vi "DriveForDistanceController.vi"(0 "Distance":dbl=60.0, 5 "Angle":dbl, 9 "SensorData":T2={"LeftDistance"=6.5916152770030445, "RightDistance"=6.599641480142774, "LeftVelocity"=46.58677937827863, "RightVelocity"=46.493891086439575, "Angle"=-0.015328918847370969, "Location"={6.595627830179985, 0.002635162832215609}}, 11 "Gains":T1={"FFV"=0.0055, "FFA"=0.0025, "Vel PID"={"P"=0.005, "I"=0.0, "D"=0.0}}, 12 "Trackwidth":dbl=30.0 format="%#_13g", 13 "Reset":bool) -> (4 "Left Speed":dbl=0.7370843765433353, 6 "Right Speed":dbl=0.7364472908610777, 10 "Done":bool, 14 "Graph":cluster{cluster{"x":dbl, "y":dbl}[]}[](graph)=[{[{"x"=0.0, "y"=0.0}, {"x"=6.0, "y"=0.0}, {"x"=12.0, "y"=0.0}, {"x"=18.0, "y"=0.0}, {"x"=24.0, "y"=0.0}, {"x"=30.0, "y"=0.0}, {"x"=36.0, "y"=0.0}, {"x"=42.0, "y"=0.0}, {"x"=48.0, "y"=0.0}, {"x"=54.0, "y"=0.0}, {"x"=55.0, "y"=0.0}, {"x"=60.0, "y"=0.0}]}, {[{"x"=6.595627830179985, "y"=0.002635162832215609}, {"x"=18.59562740071374, "y"=0.005845644049807444}]}, {[{"x"=18.595627540843186, "y"=0.0}]}, {[{"x"=18.595627830179986, "y"=0.002635162832215609}, {"x"=18.333399038985654, "y"=2.4975754526453273}, {"x"=17.558173321891196, "y"=4.883474879741818}, {"x"=16.303831762679355, "y"=7.0560581903418935}, {"x"=14.625195106486284, "y"=8.920373068560945}, {"x"=12.595627830179986, "y"=10.394940008245479}, {"x"=10.303831762679355, "y"=11.415313358374057}, {"x"=7.849969389391829, "y"=11.936897907251494}, {"x"=5.341286270968144, "y"=11.936897907251495}, {"x"=2.8874238976806166, "y"=11.415313358374059}, {"x"=0.5956278301799873, "y"=10.394940008245479}, {"x"=-1.4339394461263106, "y"=8.920373068560949}, {"x"=-3.112576102319383, "y"=7.056058190341894}, {"x"=-4.366917661531224, "y"=4.883474879741821}, {"x"=-5.142143378625682, "y"=2.497575452645332}, {"x"=-5.404372169820015, "y"=0.0026351628322170786}, {"x"=-5.142143378625684, "y"=-2.4923051269808933}, {"x"=-4.366917661531228, "y"=-4.878204554077382}, {"x"=-3.1125761023193865, "y"=-7.050787864677461}, {"x"=-1.4339394461263177, "y"=-8.915102742896513}, {"x"=0.5956278301799793, "y"=-10.389669682581046}, {"x"=2.887423897680614, "y"=-11.410043032709627}, {"x"=5.3412862709681335, "y"=-11.931627581587064}, {"x"=7.849969389391821, "y"=-11.931627581587065}, {"x"=10.303831762679351, "y"=-11.410043032709629}, {"x"=12.595627830179977, "y"=-10.389669682581053}, {"x"=14.625195106486277, "y"=-8.91510274289652}, {"x"=16.30383176267935, "y"=-7.050787864677464}, {"x"=17.558173321891193, "y"=-4.878204554077395}, {"x"=18.33339903898565, "y"=-2.492305126980903}, {"x"=18.595627830179986, "y"=0.00263516283221267}]}, {[{"x"=12326.754773558361, "y"=-12316.860814743844}, {"x"=12057.601746111126, "y"=-9756.040817653475}, {"x"=11261.905942608384, "y"=-7307.140942613652}, {"x"=9974.443087835292, "y"=-5077.189865288984}, {"x"=8251.481486477638, "y"=-3163.647148251028}, {"x"=6168.322828201805, "y"=-1650.1437904310478}, {"x"=3816.0111424787337, "y"=-602.8271511606581}, {"x"=1297.3537376183413, "y"=-67.46999315879293}, {"x"=-1277.571971927846, "y"=-67.46999315879111}, {"x"=-3796.2293767882416, "y"=-602.8271511606563}, {"x"=-6148.541062511309, "y"=-1650.143790431046}, {"x"=-8231.699720787143, "y"=-3163.647148251024}, {"x"=-9954.661322144799, "y"=-5077.189865288982}, {"x"=-11242.12417691789, "y"=-7307.14094261365}, {"x"=-12037.819980420634, "y"=-9756.04081765347}, {"x"=-12306.97300786787, "y"=-12316.860814743843}, {"x"=-12037.819980420634, "y"=-14877.68081183421}, {"x"=-11242.124176917896, "y"=-17326.580686874033}, {"x"=-9954.6613221448, "y"=-19556.531764198706}, {"x"=-8231.69972078715, "y"=-21470.07448123666}, {"x"=-6148.541062511317, "y"=-22983.57783905664}, {"x"=-3796.2293767882443, "y"=-24030.89447832703}, {"x"=-1277.5719719278572, "y"=-24566.251636328896}, {"x"=1297.3537376183326, "y"=-24566.251636328896}, {"x"=3816.011142478731, "y"=-24030.894478327034}, {"x"=6168.322828201795, "y"=-22983.57783905665}, {"x"=8251.481486477633, "y"=-21470.07448123667}, {"x"=9974.44308783529, "y"=-19556.531764198706}, {"x"=11261.90594260838, "y"=-17326.580686874047}, {"x"=12057.601746111126, "y"=-14877.68081183422}, {"x"=12326.754773558361, "y"=-12316.860814743848}]}], 15 "Time Left":dbl=20.0)   [LabVIEW 2019]
uses:
  PurePursuit/RobotNeededPathData.ctl
panel:
  in  "MaxDeAccel":dbl=120.0 format="%#_13g"
  in  "LookaheadDist":dbl=20.0
  in  "SlowSpeed":dbl=23.0 format="%#_13g"
  in  "SlowDistanceAtEnd":dbl=12.0 format="%#_13g"
  in  "MaxAccel":dbl=100.0
  in  "MaxVel":dbl=60.0
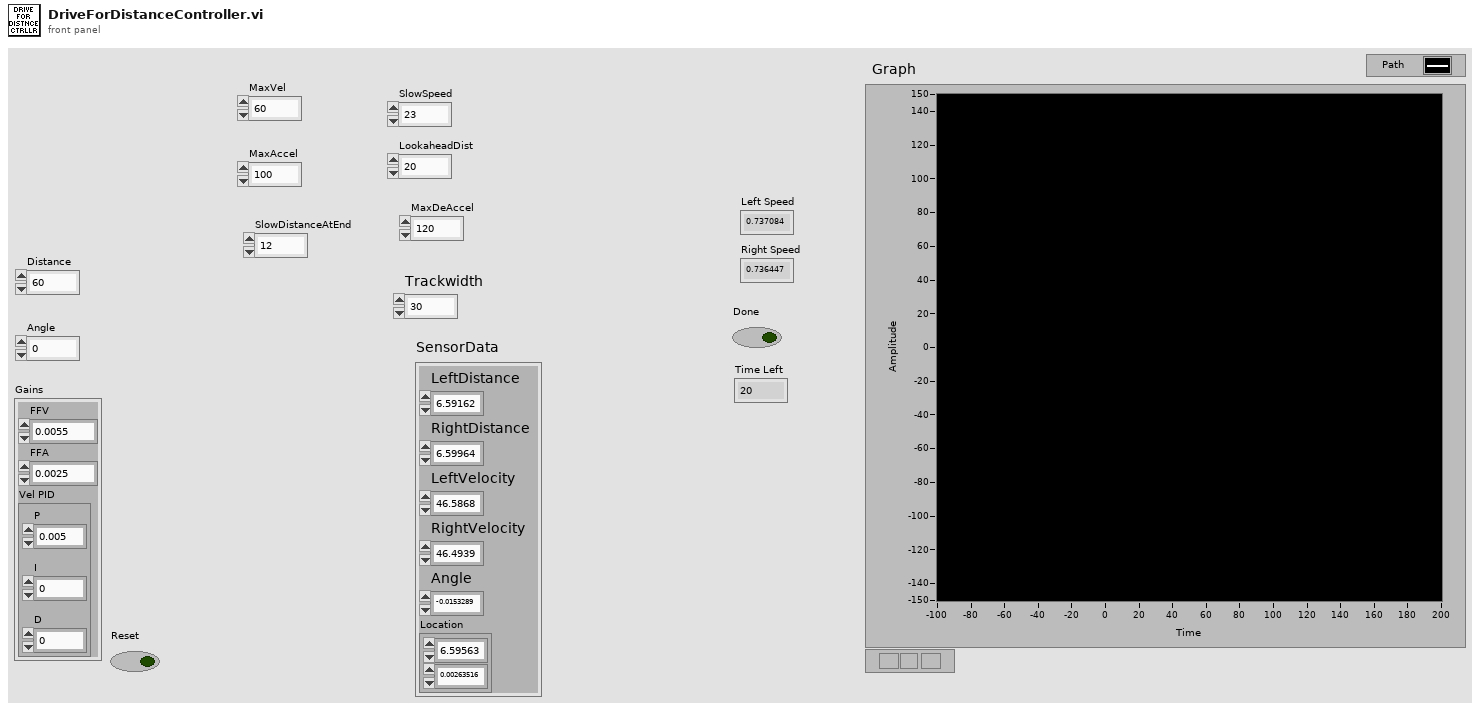
[diagram p1: front panel]
types:
  T1 = cluster{"FFV":dbl, "FFA":dbl, "Vel PID":cluster{"P":dbl, "I":dbl, "D":dbl}}
  T2 = cluster{"LeftDistance":dbl, "RightDistance":dbl, "LeftVelocity":dbl, "RightVelocity":dbl, "Angle":dbl, "Location":cluster{dbl, dbl}}
  T3 = typedef "RobotNeededPathData.ctl" = cluster{"Path":cluster{dbl, dbl}[], "MaxVel":dbl, "MaxAccel":dbl, "Backwards?":bool, "PointSpacing":dbl, "LookaheadDist":dbl, "Speed/Curve":dbl, "SlowDistanceAtEnd":dbl, "SlowSpeed":dbl, "MaxDeAccel":dbl}
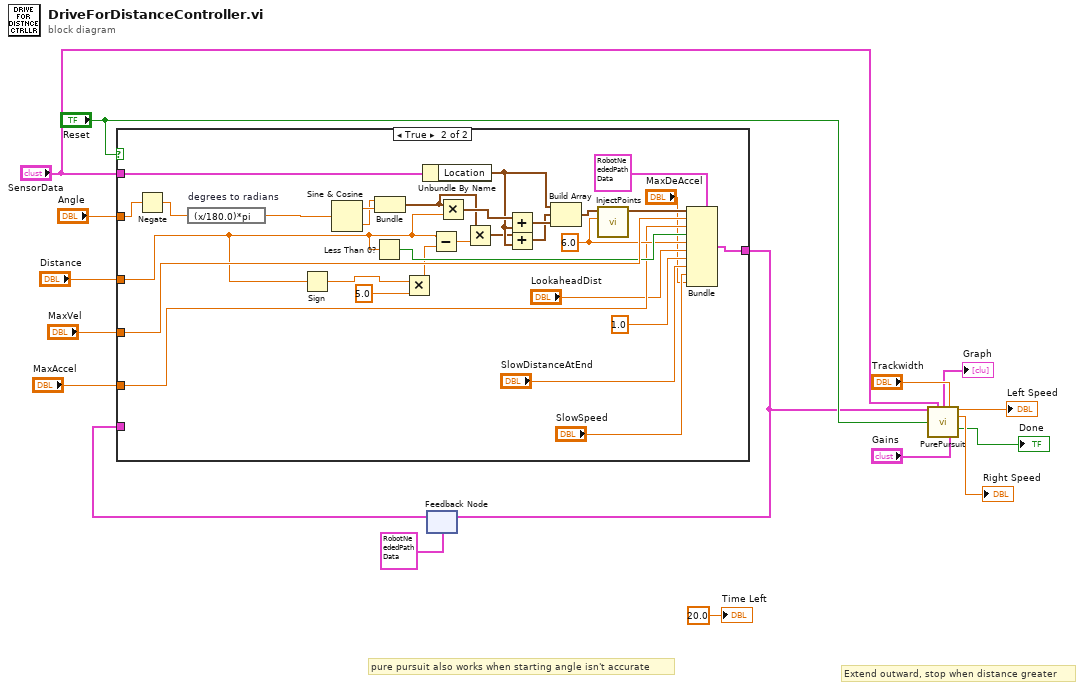
[diagram p0: block diagram]
diagram:
  # "pure pursuit also works when starting angle isn't accurate"
  # "Extend outward, stop when distance greater"
  n1 = feedback #1(T3 {"Path"=[], "MaxVel"=0.0, "MaxAccel"=0.0, "Backwards?"=FALSE, "PointSpacing"=0.0, "LookaheadDist"=0.0, "Speed/Curve"=1.8, "SlowDistanceAtEnd"=12.0, "SlowSpeed"=15.0, "MaxDeAccel"=0.0} ("RobotNeededPathData")) -> (w8:T3)
  n2 = case shown="True" "Reset" {
    tunnel: "SensorData" -> [_ w47]
    tunnel: "Angle" -> [_ w30]
    tunnel: "Distance" -> [_ w21]
    tunnel: "MaxVel" -> [_ w39]
    tunnel: "MaxAccel" -> [_ w35]
    tunnel: [w17 w31] -> w6
    tunnel: w8 -> [w17 _]
    frame False {
    }
    frame True {
      w37 = 6.0 ("Spacing")
      n3 = Negate(x=w30) -> (-x=w29:dbl)
      n4 = expression code="(x/180.0)*pi" "degrees to radians"(w29) -> (w46:dbl)
      n5 = Sign(1:w21) -> (0:w22:dbl)
      n6 = Sine & Cosine(0:w46) -> (1:w45:dbl, 2:w44:dbl)
      n7 = Less Than 0?(x=w21) -> (x < 0?=w38:bool)
      n8 = Bundle(w44, w45) -> (w28:cluster{dbl, dbl})  [unwired: 1 in]
      n9 = Multiply(x=w22, y=5.0) -> (x*y=w20:dbl)
      n10 = Unbundle By Name(w47) -> ("Location"=w27:cluster{dbl, dbl})
      n11 = Subtract(x=w21, y=w20) -> (x-y=w25:dbl)
      n12 = Multiply(x=w28, y=w21) -> (x*y=w43:cluster{dbl, dbl})
      n13 = Multiply(x=w28, y=w25) -> (x*y=w26:cluster{dbl, dbl})
      n14 = Add(x=w43, y=w27) -> (x+y=w19:cluster{dbl, dbl})
      n15 = Add(x=w26, y=w27) -> (x+y=w18:cluster{dbl, dbl})
      n16 = Build Array(w27, w18, w19) -> (w42:cluster{dbl, dbl}[])
      n17 = call "InjectPoints.vi"("Spacing"=w37, "Path"=w42) -> ("Path out"=w40:cluster{dbl, dbl}[])  [unwired: 9 in]
      n18 = Bundle(cluster=T3 {"Path"=[], "MaxVel"=0.0, "MaxAccel"=0.0, "Backwards?"=FALSE, "PointSpacing"=0.0, "LookaheadDist"=0.0, "Speed/Curve"=1.8, "SlowDistanceAtEnd"=12.0, "SlowSpeed"=15.0, "MaxDeAccel"=0.0} ("RobotNeededPathData"), "Path"=w40, "MaxVel"=w39, "MaxAccel"=w35, "Backwards?"=w38, "PointSpacing"=w37, "LookaheadDist"="LookaheadDist", "Speed/Curve"=1.0, "SlowDistanceAtEnd"="SlowDistanceAtEnd", "SlowSpeed"="SlowSpeed", "MaxDeAccel"="MaxDeAccel") -> (w31:T3)
    }
  }
  n19 = feedback-in #1(w6) -> ()
  n20 = call "PurePursuit.vi"("RobotNeededPathData"=w6, "SensorData"="SensorData", "Trackwidth"="Trackwidth", "Reset"="Reset", "Gains"="Gains") -> ("Graph"=→"Graph":cluster{cluster{"x":dbl, "y":dbl}[]}[], "LeftValue"=→"Left Speed":dbl, "RightValue"=→"Right Speed":dbl, "Done"=→"Done":bool)  [unwired: 5 in, 2 out]
  "Time Left" <- 20.0 ("Time Left")
